vi "Log50mA.vi"(7 "Area":i32, 8 "error in (no error)":errorcluster, 9 "Reverse":dbl, 10 "50mA Data":T1 {"Reverse" format="%#_3g"; "Current,mA" format="%_6g"; "Knee Current" format="%#_3g"; "WL" format="%_6g"; "Voltage" format="%_6g"; "Power" format="%_5g"}, 11 "LotData in":refnum<class "LotData.lvclass">) -> (0 "error out":errorcluster, 3 "LotData out":refnum<class "LotData.lvclass">)   [LabVIEW 2012, in "LotData.lvclass"]
uses:
  LotData.lvclass
  Controls/Measurement.ctl
  <vilib>/addons/database/Auxilliary.llb/DB Tools Parameter Info.ctl
  <vilib>/addons/database/Auxilliary.llb/DB Tools DataTypes.ctl
  <vilib>/addons/database/Auxilliary.llb/DB Tools Parameter Dir.ctl
  LotData.lvclass/LotData.ctl
  <vilib>/addons/database/Connection.llb/DB Tools Open Connec (Path).vi
  <vilib>/addons/database/Command.llb/Cmd Set Parameter Value (C).vi
  <vilib>/addons/database/Command.llb/Cmd Execute.vi
  <vilib>/addons/database/Recordset.llb/Rec Destroy - Command.vi
  <vilib>/addons/database/Command.llb/Cmd Delete.vi
  <vilib>/addons/database/NI_Database_API.lvlib
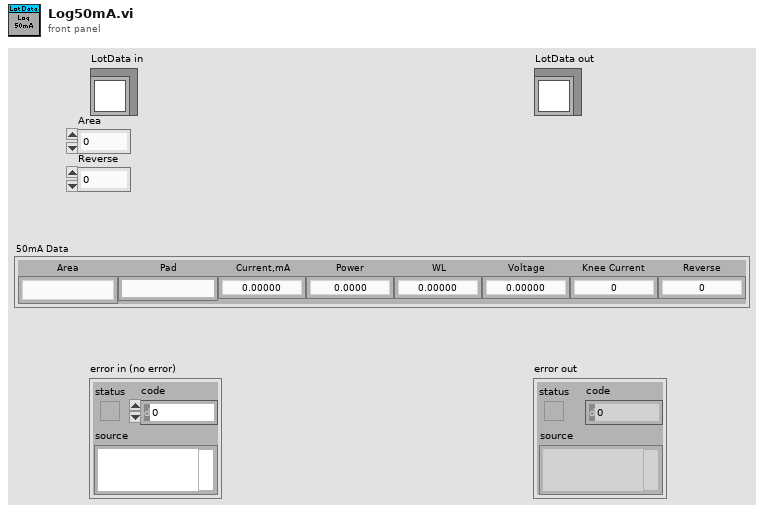
[diagram p1: front panel]
types:
  T1 = typedef "Measurement.ctl" = cluster{"Area":string, "Pad":string, "Current,mA":dbl, "Power":dbl, "WL":dbl, "Voltage":dbl, "Knee Current":dbl, "Reverse":dbl}
  T2 = typedef "NI_Database_API.lvlib/DB Tools Parameter Info.ctl" = cluster{"parameter name":string, "type":T3, "direction":T4, "value":variant}
  T3 = typedef "NI_Database_API.lvlib/DB Tools DataTypes.ctl" = enum16{"String", "Long (I32)", "Single (SGL)", "Double (DBL)", "Date/Time", "Binary"}
  T4 = typedef "NI_Database_API.lvlib/DB Tools Parameter Dir.ctl" = enum32{"Input", "Output", "Input/Output", "Return Value"}
  T5 = typedef "NI_Database_API.lvlib/Conn ObjectReference.ctl" = refnum<k1>
  T6 = typedef "NI_Database_API.lvlib/Cmd ObjectReference.ctl" = refnum<k1>
  T7 = typedef "NI_Database_API.lvlib/Cmd-Rec Object Reference.ctl" = refnum<k1>
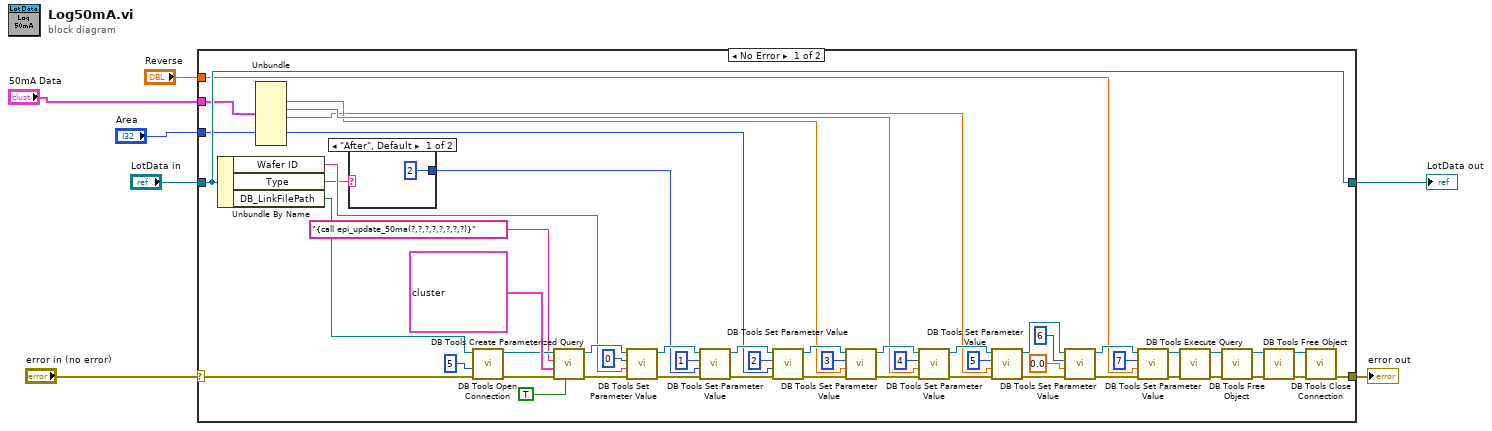
[diagram p0: block diagram]
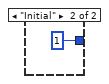
[diagram p2: hidden frame]
diagram:
  n1 = case shown="No Error" "error in (no error)" {
    selector: "error in (no error)" -> [w22 w63]
    tunnel: [w18 w63] -> w6
    tunnel: [w17 w62] -> w4
    tunnel: "LotData in" -> [w17 w62]
    tunnel: "50mA Data" -> [w16 _]
    tunnel: "Area" -> [w15 _]
    tunnel: "Reverse" -> [w10 _]
    frame No Error {
      n2 = Unbundle By Name(w17) -> ("Wafer ID"=w21:string, "Type"=w20:string, "DB_LinkFilePath"=w9:path)
      n3 = Unbundle(w16) -> ("Current,mA"=w13:dbl, "Power"=w14:dbl, "WL"=w12:dbl)  [unwired: 5 out]
      n4 = case shown="\"After\", Default" w20 {
        tunnel: [2 1] -> w19
        frame "After", Default {
        }
        frame "Initial" {
        }
      }
      n5 = call-poly <vilib>:"DB Tools Open Connection.vi"("error in (no error)"=w22, "connection timeout (15)"=5, "connection information"=w9) -> ("error out"=w56:errorcluster, "connection reference"=w57:T5)  [unwired: 5 in]
      n6 = call <vilib>:"DB Tools Create Parameterized Query.vi"("stored procedure? (F)"=TRUE, "error in (no error)"=w56, "parameters"=T2[] [{"parameter name"="wafer", "type"=enum."String", "direction"=enum."Input", "value"=variant}, {"parameter name"="test", "type"=enum."Single (SGL)", "direction"=enum."Input", "value"=variant}, {"parameter name"="area", "type"=enum."Single (SGL)", "direction"=enum."Input", "value"=variant}, {"parameter name"="wl", "type"=enum."Double (DBL)", "direction"=enum."Input", "value"=variant}, {"parameter name"="power", "type"=enum."Double (DBL)", "direction"=enum."Input", "value"=variant}, {"parameter name"="voltage", "type"=enum."Double (DBL)", "direction"=enum."Input", "value"=variant}, {"parameter name"="knee", "type"=enum."Double (DBL)", "direction"=enum."Input", "value"=variant}, {"parameter name"="reverse", "type"=enum."Double (DBL)", "direction"=enum."Input", "value"=variant}], "SQL query"="{call epi_update_50ma(?,?,?,?,?,?,?,?)}", "connection reference"=w57) -> ("error out"=w53:errorcluster, "command reference"=w52:T6)  [unwired: 2 in, 1 out]
      n7 = call-poly <vilib>:"DB Tools Set Parameter Value.vi"("error in (no error)"=w53, "value"=w21, "parameter index"=0, "command reference"=w52) -> ("error out"=w23:errorcluster, "command reference out"=w38:T6)  [unwired: 4 in]
      n8 = call-poly <vilib>:"DB Tools Set Parameter Value.vi"("error in (no error)"=w23, "value"=w19, "parameter index"=1, "command reference"=w38) -> ("error out"=w24:errorcluster, "command reference out"=w37:T6)  [unwired: 4 in]
      n9 = call-poly <vilib>:"DB Tools Set Parameter Value.vi"("error in (no error)"=w24, "value"=w15, "parameter index"=2, "command reference"=w37) -> ("error out"=w25:errorcluster, "command reference out"=w36:T6)  [unwired: 4 in]
      n10 = call-poly <vilib>:"DB Tools Set Parameter Value.vi"("error in (no error)"=w25, "value"=w13, "parameter index"=3, "command reference"=w36) -> ("error out"=w26:errorcluster, "command reference out"=w35:T6)  [unwired: 4 in]
      n11 = call-poly <vilib>:"DB Tools Set Parameter Value.vi"("error in (no error)"=w26, "value"=w14, "parameter index"=4, "command reference"=w35) -> ("error out"=w27:errorcluster, "command reference out"=w34:T6)  [unwired: 4 in]
      n12 = call-poly <vilib>:"DB Tools Set Parameter Value.vi"("error in (no error)"=w27, "value"=w12, "parameter index"=5, "command reference"=w34) -> ("error out"=w28:errorcluster, "command reference out"=w33:T6)  [unwired: 4 in]
      n13 = call-poly <vilib>:"DB Tools Set Parameter Value.vi"("error in (no error)"=w28, "value"=0.0, "parameter index"=6, "command reference"=w33) -> ("error out"=w29:errorcluster, "command reference out"=w32:T6)  [unwired: 4 in]
      n14 = call-poly <vilib>:"DB Tools Set Parameter Value.vi"("error in (no error)"=w29, "value"=w10, "parameter index"=7, "command reference"=w32) -> ("error out"=w30:errorcluster, "command reference out"=w31:T6)  [unwired: 4 in]
      n15 = call-poly <vilib>:"DB Tools Execute Query.vi"("error in (no error)"=w30, "command reference"=w31) -> ("error out"=w49:errorcluster, "command-recordset reference"=w50:T7)  [unwired: 6 in]
      n16 = call-poly <vilib>:"DB Tools Free Object.vi"("error in (no error)"=w49, "command-recordset reference"=w50) -> ("error out"=w51:errorcluster, "command reference"=w48:T6)  [unwired: 8 in]
      n17 = call-poly <vilib>:"DB Tools Free Object.vi"("error in (no error)"=w51, "command reference"=w48) -> ("error out"=w46:errorcluster, "connection reference"=w47:T5)  [unwired: 8 in]
      n18 = call <vilib>:"DB Tools Close Connection.vi"("error in (no error)"=w46, "connection reference"=w47) -> ("error out"=w18:errorcluster)  [unwired: 5 in]
    }
    frame Error {
    }
  }
  "error out" <- w6
  "LotData out" <- w4
